vi "SetCalibrationWidgetsVisibility.vi"(10 "show":bool, 11 "ReferencesCluster":T1) -> ()   [LabVIEW 2013]
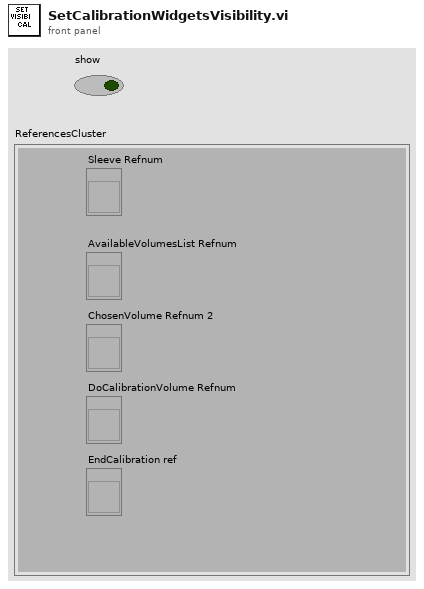
[diagram p1: front panel]
types:
  T1 = cluster{"Sleeve Refnum":refnum<vi>, "AvailableVolumesList Refnum":refnum<vi>, "ChosenVolume Refnum 2":refnum<vi>, "DoCalibrationVolume Refnum":refnum<vi>, "EndCalibration ref":refnum<vi>}
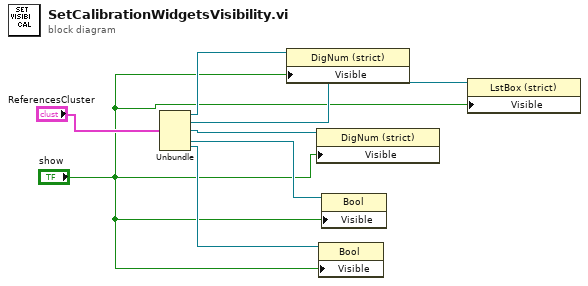
[diagram p0: block diagram]
diagram:
  n1 = Unbundle("ReferencesCluster") -> ("Sleeve Refnum"=w6:refnum<vi>, "AvailableVolumesList Refnum"=w5:refnum<vi>, "ChosenVolume Refnum 2"=w4:refnum<vi>, "DoCalibrationVolume Refnum"=w3:refnum<vi>, "EndCalibration ref"=w2:refnum<vi>)
  n2 = property class="DigNum (strict)"(reference=w6, "Visible"="show") -> ()  [unwired: 1 in, 2 out]
  n3 = property class="DigNum (strict)"(reference=w4, "Visible"="show") -> ()  [unwired: 1 in, 2 out]
  n4 = property class="Bool"(reference=w2, "Visible"="show") -> ()  [unwired: 1 in, 2 out]
  n5 = property class="Bool"(reference=w3, "Visible"="show") -> ()  [unwired: 1 in, 2 out]
  n6 = property class="LstBox (strict)"(reference=w5, "Visible"="show") -> ()  [unwired: 1 in, 2 out]
